vi "Forebrain - Bill.vi"() -> ()   [LabVIEW 2012]
doc: "This VI contrains the Forebrain within the Olin Robot Architecture. It must be run first to load the appropriate mission definition files. It contains a finite state machine built around a tabbed Operator interface that will guide an operator through the startup, run shutdown mission sequence. After running it, run the Midbrain and Hindbrain VIS."
panel:
  out "Number Waypoints":i32
  out "NXT String Sent":string="$B^"
  in  "Soft E-Stop":bool
  out "NXT String Received":string
  out "return count":u32
  out "error out":errorcluster
  in  "error in 2":errorcluster
  out "Desired \nVelocity":i16=5
  out "Local\nHeading":i16=90
  out "Ycurrent":dbl format="%#_3g"
  out "Xcurrent":dbl format="%#_3g"
  out "Ystart":dbl
  out "Xstart":dbl
  in  "error in":errorcluster
  out "Robot Live":bool
  in  "E-Stop":bool
  in  "Tab":T1(tab)
  out "MissionTime (Min)":dbl(knob) scale=0.0..10.0
  out "LidarDist":i16
  out "IR Index":i32
  out "BatteryLevel":dbl(slide) scale=6.0..9.0
  out "String Received":string
  out "Send String":string="$B^"
  in  "VISA resource name":refnum<visa-resource-name>="COM6"
  in  "Mode":i16 min=0 max=99 step=1
  in  "Desired Vel":i16(slide)=7 scale=0.0..14.0
  in  "Local Head":i16(slide)=7 scale=0.0..14.0
  out "StartMissionMap":picture
  out "MapDARCheck":picture
  in  "RunRobot":bool
  in  "Tug letter":string="G"
  out "Tug X":i32
  out "Tug Y":i32
  out "Tug H":i32
  out "BS Time Out?":bool
  out "Buoy locations":cluster{"regular expression":string, i32, i32}[](array[cluster])
  out "Valid ?":bool
  out "Battery\nVolts":i16
  out "Base Station data rec'd":string
  out "udp rate":bool
  out "CollisionWarning":bool
  out "DebugMapDAR":picture
  in  "MapDAR Control":T2={"NumberOfBeams"=180, "SensorRange"=500.0, "Noise (0.1 to 1)"=0.0} {"Noise (0.1 to 1)" min=0.0 max=1.0 step=0.1; "SensorRange" min=500.0 max=1500.0 step=100.0; "NumberOfBeams" min=36 max=360 step=2}
  out "MapDAR Data (r:pixel b:degrees)":cluster{"Range":dbl, "Bearing":dbl}[](array[cluster])
  in  "Stop DebugSENSE":bool
  out "MissionMap":picture
  out "Tug position":T3
  out "initialized MDF":T4(array[cluster])
  out "Way Point Index":i32
  out "InitialWaypoint":cluster{"X":i16, "Y":i16}
  in  "Pen Color":u32(colorbox)=15671808
  in  "Select Pen Attributes":T5={"Width"=1, "Style"=enum."Solid"}
  out "Draw??":bool
  in  "WhereAmI?FromBase":T6
  out "(xr,yr)":cluster{"X":dbl, "Y":dbl}
  in  "RobotPosition":T3 {"xrobot" min=0.0 max=1177.0 step=10.0; "yrobot" min=0.0 max=850.0 step=10.0; "heading" min=0.0 max=7.0 step=0.1}
  out "MDF_Original":T4(array[cluster])
  out "WhatAroundMeMap?":cluster{"T":dbl, "Range":dbl, "Bearing":dbl}[](array[cluster])
  out "WayPointAct":dbl[](array[numeric])
  out "SteerAngle":dbl
  out "MissionDefFile":picture
  out "MDF":T4(array[cluster])
  in  "Select Your Behavior":T7(ring)
  out "No. of Waypoints":i32
  in  "Exit Planning":bool
  in  "BoatSpeed for Leg":dbl(slide)=8.0 min=-9.0 max=9.0 step=1.0 scale=0.0..14.0
  out "BuildMDF":bool
  out "WayPoint Position":cluster{"X":i32, "Y":i32}
  in  "Upper Midbrain Active":bool
  out "Send String to NXT":string="$B^"
  in  "Behavior Command":T7(ring)
  out "CollisionLight":bool
  out "Where? Manual":T6
  out "ActManual":bool
  in  "Manual Heading":i16(knob) min=0 max=14 step=1
  out "MWhat?":bool
  out "Where? 2":bool
  out "How? 2":bool
  in  "ManualModeStop":bool
  out "ManualModeMapDAR":picture
  out "ManualMissionMap":picture
  out "Battery":dbl(slide) scale=0.0..8.0
  in  "Manual Vel":dbl(slide) min=0.0 max=14.0 step=1.0 scale=0.0..14.0
  out "MissionTime":dbl(knob) scale=0.0..10.0
  out "Heading":cluster{dbl, dbl}(knob)={0.0, 34.390870865624734} scale=180.0..-179.0 scale format="%#_3g"
  out "Speed":i16(knob) scale=-6.0..6.0
  out "Current Behavior":T7(ring)
  out "Robot Position":cluster{"X":dbl, "Y":dbl} {"X" format="%#_3g"; "Y" format="%#_3g"}
  out "Ready":bool
  in  "Pause":bool
  in  "Rerun MDF":bool
  out "CollisionLight 2":bool
  out "Act":bool
  out "Neo-C":bool
  out "How?":bool
  out "What?":bool
  out "A Heading":cluster{dbl, dbl}(knob)={0.0, 34.390870865624734} scale=180.0..-180.0
  out "A Speed":dbl(knob) scale=-9.0..9.0
  out "AutoBattery":dbl(slide) scale=0.0..8.0
  out "AutoModeLIDAR":picture
  out "AutoMissionMap":picture
  in  "RunAutoMode":bool
  out "MissionTimeAuto":dbl(knob) scale=0.0..60.0
  out "Where?":bool
  out "Current Waypoint":dbl
  in  "Manual Override":bool
  in  "Destinations Array":i64[][](array[numeric])
  out "BAM Mission Map":picture
  in  "Pixel Y Goal":dbl
  in  "Pixel X Goal":dbl
  out "Pixel X":dbl
  out "Pixel Y":dbl
  out "Direction":dbl
  out "Base Station String":string
  out "Battery Level":dbl
  in  "Heading":i16(knob)=7
  in  "Velocity":i16(slide)=7 scale=0.0..14.0
  # "To run\nrobot,\nclick\narrow\nabove\n\nRun Robot button must be on"
  # "Operation Directions\n\n1)Click on Startup&\nShutdown tab.\n2) Click on Run \nArrow on menubar.\nRun Forebrain,\nvis from the project\nexplorer.\n3) Select a mssion \nmap file when asked.\n4) Check robot is \nfully operational on\nStartup tab.\n5) Debug with debug\ntabs as required.\n6) Select ManualMode\ntab and test drive \nrobot.\n7) Select PlanMission\ntab and set up \nmission.\n8) Go to AutoMode\ntab and run mission."
  # "Turns off drive\nmotors"
  # "Enter Olin Test  Pool"
  # "Xbee Com Port"
  # "xBee\"Send String\" (mode, desired velocity, local heading)"
  # "(Type in Tug Letter  L T G P  (look at boat cradle)"
  # "Should be on to\nrun"
  # "BoatG,X,Y,H,BoatT,X,Y,H,BoatP,X,Y.H,BoatL,X,Y,H,BuoyA,X,Y,BuoyB,X,Y,BuoyC,X,Y,BuoyD,X,Y,Time(hours,Min,Sec)"
  # "To stop  program \nturn off here"
  # "Use this tab\nto explore\nLIDAR\ndata and \noperation"
  # "Set\nNumberOfBeams\nSensorRange\nNoise\nto\nview\nsimulated\nsensor\ndata"
  # "Turn Debug Sim \nto leave this\ntab--->"
  # "This tab will auto\nreturn to Startup \nin 2 seconds"
  # "Clean up interface and make more useful for debugging behaviors"
  # "Build out interface and make more useful for debugging act"
  # "This tab will auto\nreturn to Startup \nin 2 seconds"
  # "Directions:\n1) Select Robot Behavior for each mission leg.\n2) Select Robot Speed for leg.\n3) Click on robots current location for first waypoint.\n4) Hold down button and drag to next\nwaypoint. Click on next leg waypoint.\n5) Hold mouse button down and drag to \nnext waypoint. \n6) Click on next waypoint. Repeat for full mission.\n7) MDF will store up to 20 waypoints."
  # "Remember to\nset boat\nleg speed !"
  # "Please Adjust Scroll Barrs in Tug Off Mode to Prevent  Extra Lines Being Drawn"
  # "\"Send String\" (mode, desired velocity, local heading)"
  # "Press to stop and return to StartUp"
  # "Open MidBrain\nArbiter to see\nBrain Waves"
  # "AutoMode\nAutomatically \nReturns to \nStartUp Mode"
  # "Pixel coordinates for destinations."
  # "BoatG,X,Y,H,BoatT,X,Y,H,BoatP,X,Y.H,BoatL,X,Y,H,BuoyA,X,Y,BuoyB,X,Y,BuoyC,X,Y,BuoyD,X,Y,Time(hours,Min,Sec)"
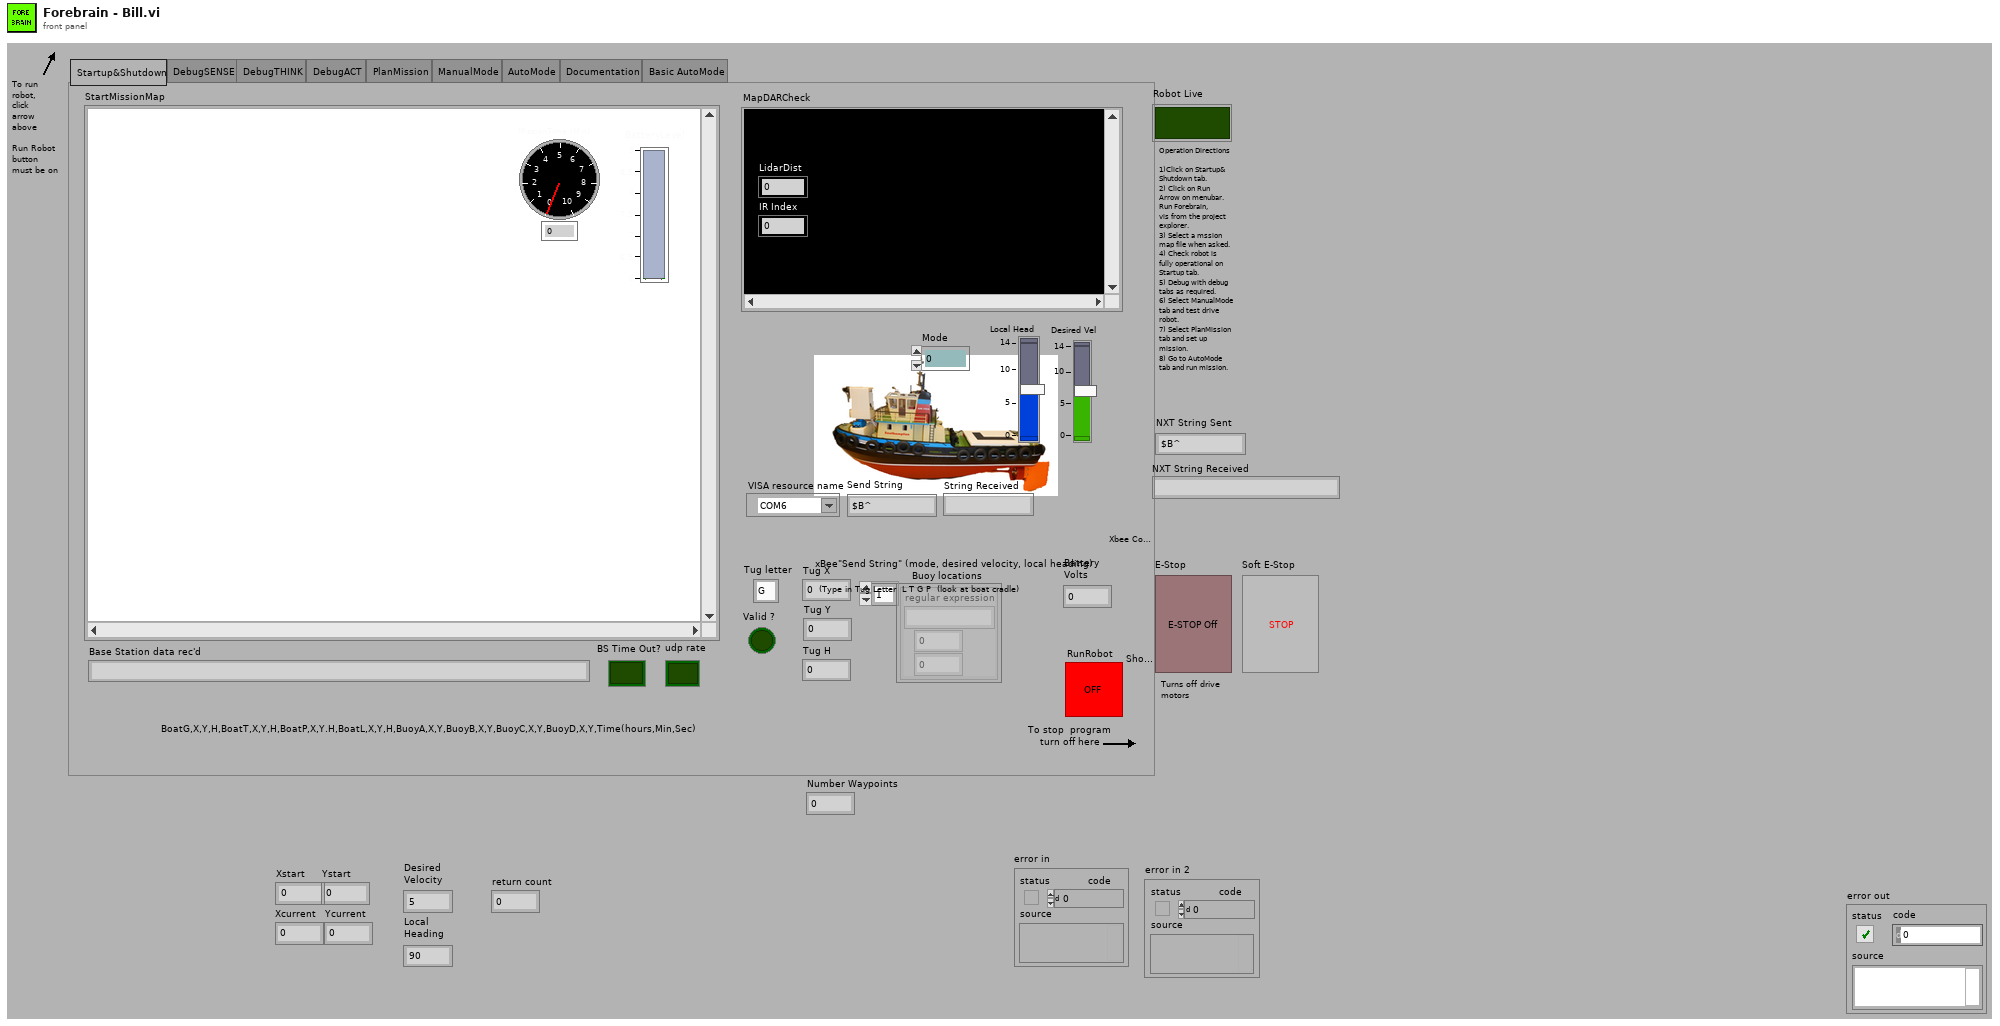
[diagram p1: front panel]
types:
  T1 = enum32{"Startup&Shutdown", "DebugSENSE", "DebugTHINK", "DebugACT", "PlanMission", "ManualMode", "AutoMode", "Documentation", "Basic AutoMode"}
  T2 = cluster{"NumberOfBeams":i32, "SensorRange":dbl, "Noise (0.1 to 1)":dbl}
  T3 = cluster{"xrobot":dbl, "yrobot":dbl, "heading":dbl}
  T4 = cluster{"Status":enum16{"Past", "Current", "Future"}, "x":dbl, "y":dbl, "z":dbl, "Vel":dbl, "Dwell Time":dbl, "BehCom":enum16{"Tug Off", "Manual Mode", "Goto WayPoint", "Back Up", "Circle", "Left Wall Follow", "Right Wall Follow", "Hunt"}, "Expand1":dbl, "Expand2":dbl, "Expand3":dbl}[]
  T5 = cluster{"Width":u16, "Style":enum32{"Solid", "Dash", "Dot", "DashDot", "DashDotDot"}}
  T6 = cluster{"T":dbl, "X":dbl, "Y":dbl, "Direction":dbl}
  T7 = enum16{"Tug Off", "Manual Mode", "Goto WayPoint", "Back Up", "Circle", "Left Wall Follow", "Right Wall Follow", "Hunt"}
  T8 = enum32{"Startup&Shutdown", "DebugSENSE", "DebugTHINK", "DebugACT", "PlanMission", "ManualMode", "AutoMode", "Documentation"}
  T9 = cluster{"VelCom":dbl, "BehCom":enum16{"OpenFieldTransit", "P-WallFollow", "S-WallFollow", "LaneFollow", "ManualMode"}}
  T10 = typedef "IMAQ Image.ctl" = refnum<image>
  T11 = typedef "imagedata.ctl" = cluster{"image type":i32, "image depth":i32, "image":u8[], "mask":u8[], "colors":u32[], "Rectangle":cluster{"left":i16, "top":i16, "right":i16, "bottom":i16}}
  T12 = cluster{"Status":enum16{"Past", "Current", "Future"}, "x":dbl, "y":dbl, "z":dbl, "Vel":dbl, "Dwell Time":dbl, "BehCom":enum16{"Tug Off", "Manual Mode", "Goto WayPoint", "Back Up", "Circle", "Left Wall Follow", "Right Wall Follow", "Hunt"}, "Expand1":dbl, "Expand2":dbl, "Expand3":dbl}
  T13 = typedef "LVMouseTypeDef.ctl" = cluster{"Mouse Position":cluster{"X":i32, "Y":i32}, "Mouse Modifiers":cluster{"Button Down":bool, "Shift Mod":bool, "Menu Mod":bool, "Option Mod":bool}}
  T14 = cluster{"regular expression":string, i32, i32, i32}
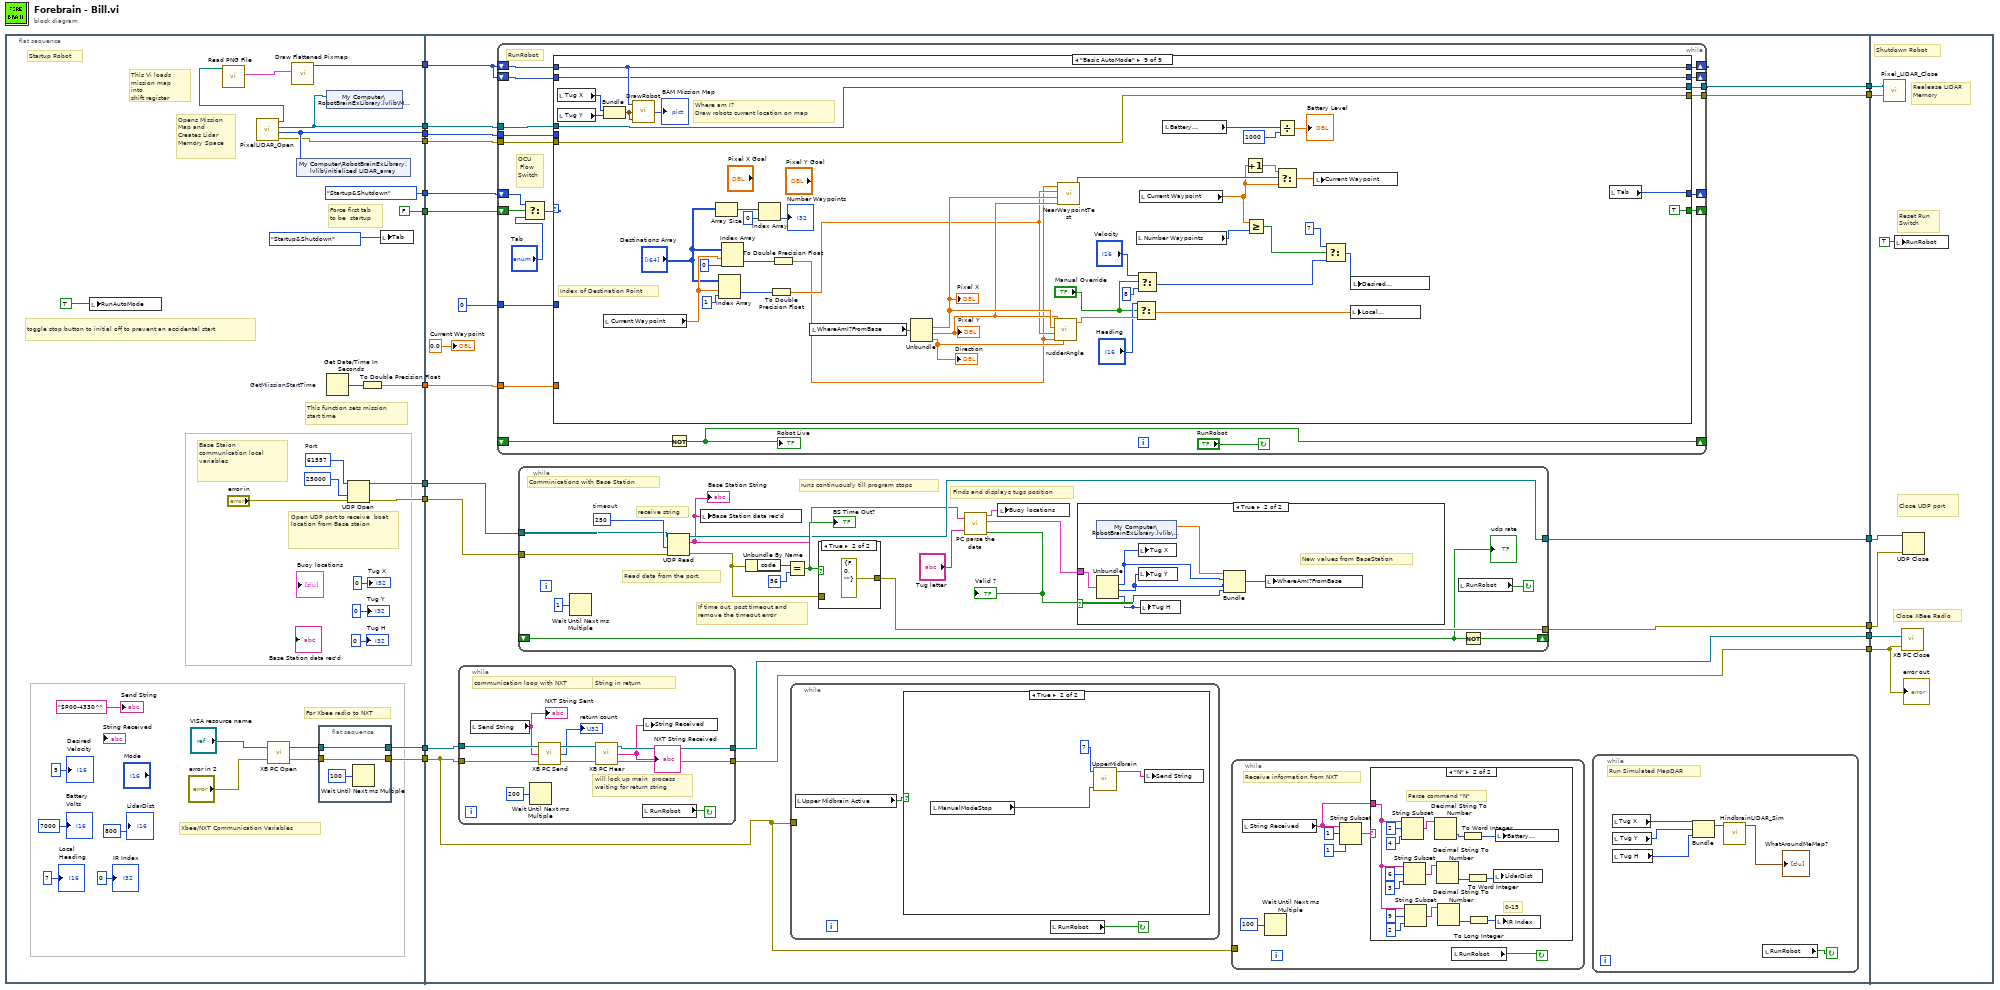
[diagram p0: block diagram]
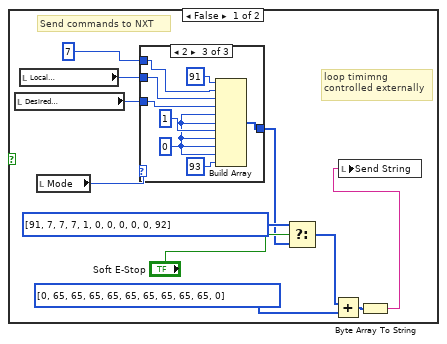
[diagram p3: hidden frame]
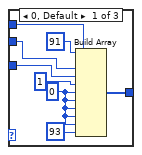
[diagram p4: hidden frame]
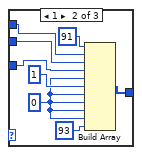
[diagram p5: hidden frame]
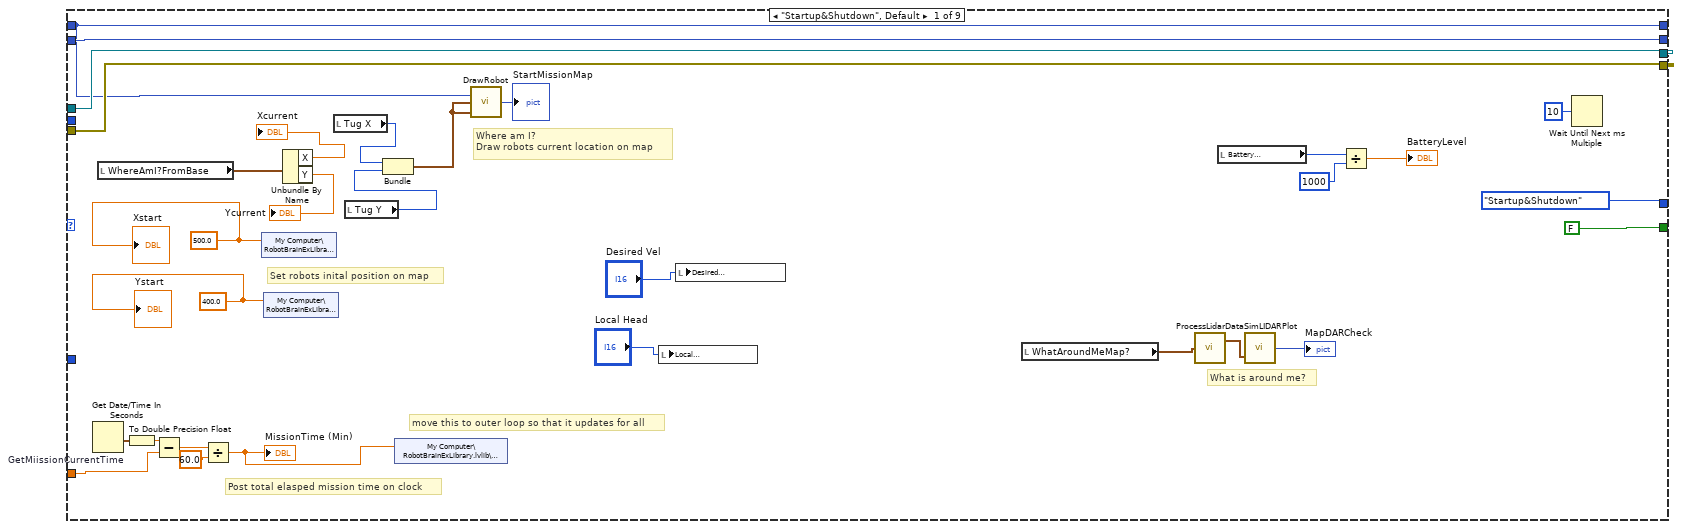
[diagram p8: hidden frame]
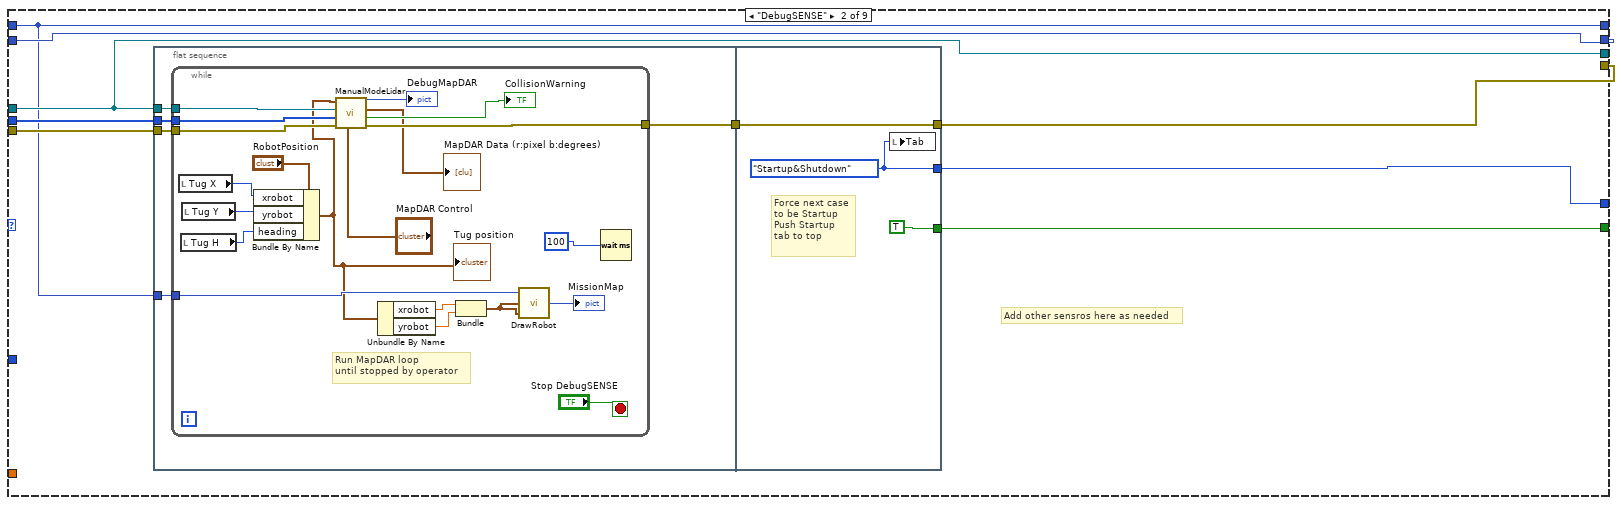
[diagram p9: hidden frame]
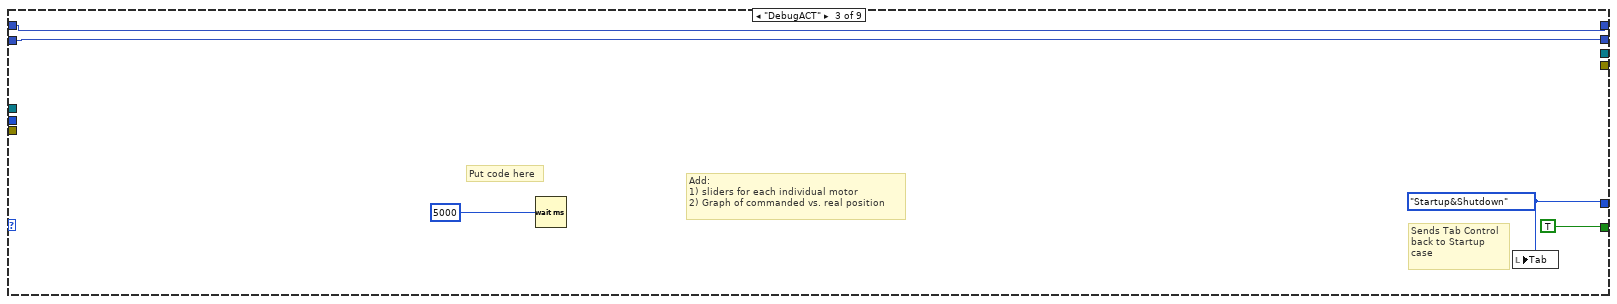
[diagram p10: hidden frame]
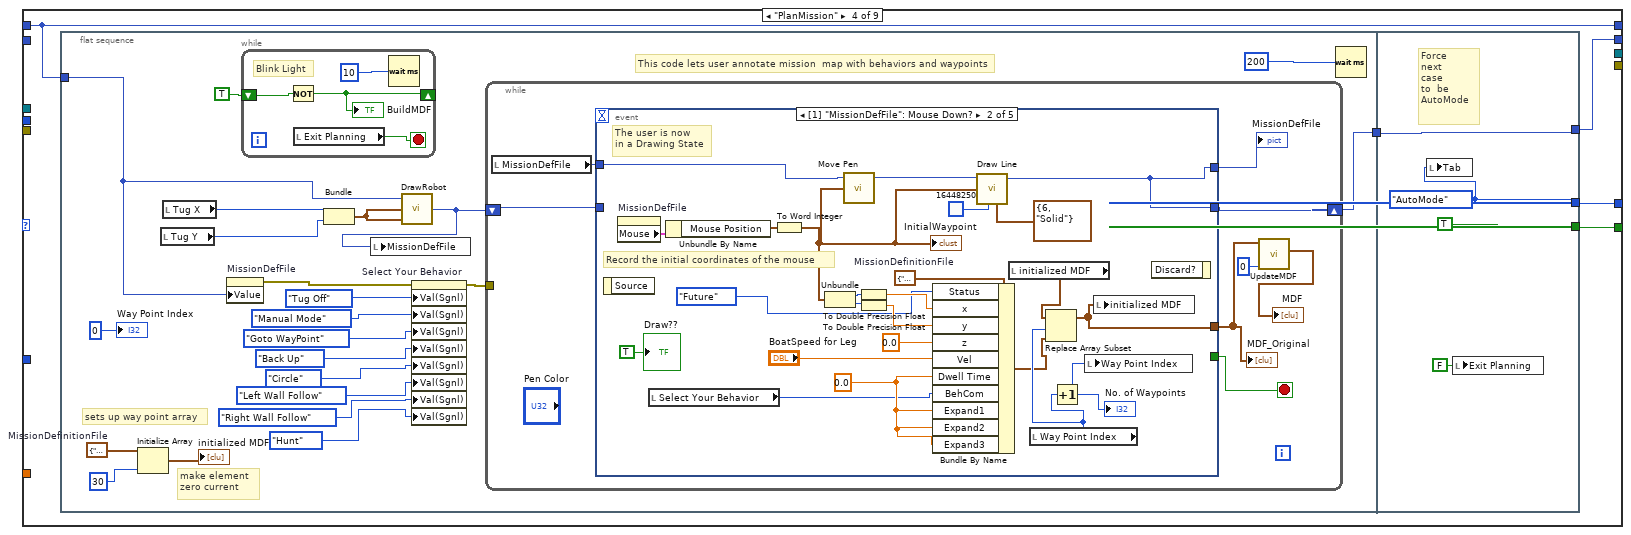
[diagram p11: hidden frame]
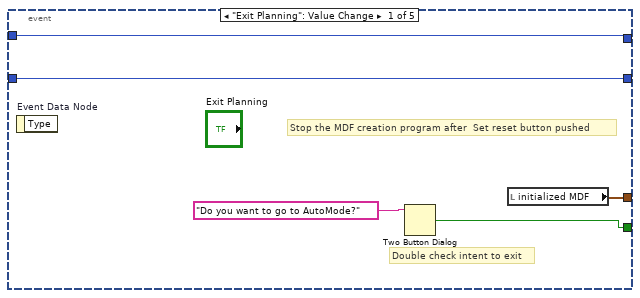
[diagram p12: hidden frame]
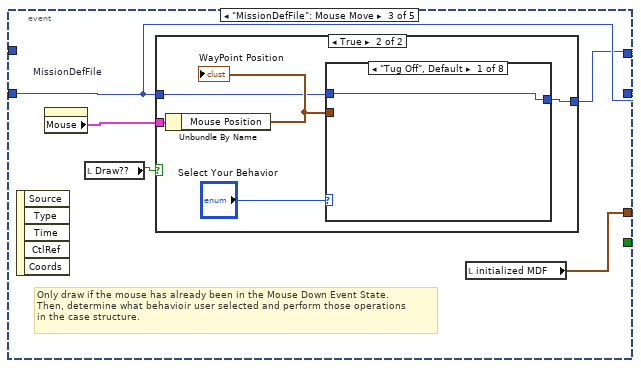
[diagram p13: hidden frame]
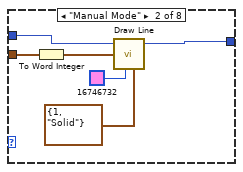
[diagram p15: hidden frame]
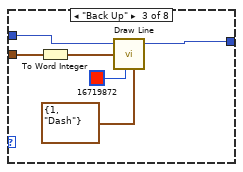
[diagram p16: hidden frame]
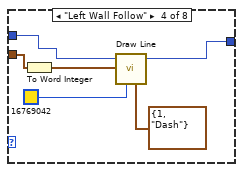
[diagram p17: hidden frame]
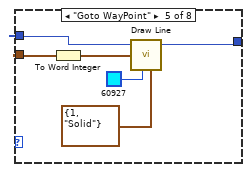
[diagram p18: hidden frame]
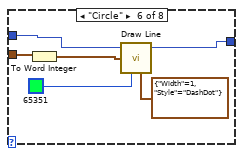
[diagram p19: hidden frame]
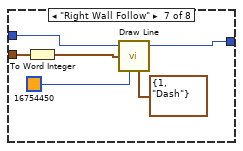
[diagram p20: hidden frame]
diagram:
  n1 = flat-sequence {
    tunnel: [w48] -> w17
    tunnel: [w47] -> w16
    tunnel: [w44] -> w15
    tunnel: [w46] -> w14
    tunnel: [w45] -> w13
    tunnel: [FALSE ("RunAutoMode")] -> w10
    tunnel: [T8."Startup&Shutdown" ("Tab")] -> w9
    tunnel: [w31] -> w8
    tunnel: [w30] -> w7
    tunnel: [w19] -> w6
    tunnel: [w18] -> w5
    tunnel: w17 -> [w71]
    tunnel: w16 -> [w70]
    tunnel: w15 -> [w69]
    tunnel: w14 -> [w68]
    tunnel: w13 -> [w67]
    tunnel: [w66] -> w12
    tunnel: [w65] -> w11
    tunnel: w10 -> [w64]
    tunnel: w9 -> [w63]
    tunnel: w8 -> [w58]
    tunnel: w7 -> [w57]
    tunnel: w6 -> [w62]
    tunnel: w5 -> [w59]
    tunnel: [w61] -> w4
    tunnel: [w60] -> w3
    tunnel: [w56] -> w2
    tunnel: [w55] -> w1
    tunnel: w12 -> [w662]
    tunnel: w11 -> [w661]
    tunnel: w4 -> [w660]
    tunnel: w3 -> [w659]
    tunnel: w2 -> [w658]
    tunnel: w1 -> [w657]
    frame #0 {
      w37 = u16 61557  # Port
      # "For Xbee radio to NXT"
      # "Xbee/NXT Communication Variables"
      # "Base Staion communication local variables"
      # "Open UDP port to receive  boat location from Base staion"
      # "Force first tab\nto be  startup"
      # "toggle stop button to initial off to prevent an accidental start"
      # "Opens Mission\nMap and\nCreates Lidar\nMemory Space"
      # "This function sets mission \nstart time"
      # "This Vi loads\nmission map into \nshift register"
      # "Startup Robot"
      n2 = local write "RunAutoMode"(TRUE ("RunAutoMode")) -> ()
      n3 = call "PixelLIDAR_Open.vi"() -> ("error out"=w45:errorcluster, "initialized LIDAR\narray"=w46:i32[], "MDF Image"=w44:T10, "MissionMap"=w39:path)  [unwired: 2 in]
      n4 = call <vilib>:"Read PNG File.vi"("path to PNG file"=w39) -> ("image data"=w38:T11)  [unwired: 8 in, 2 out]
      n5 = call "XB PC Open.vi"("error in (no error)"="error in 2", "VISA resource name"="VISA resource name") -> ("error out"=w22:errorcluster, "VISA resource name out"=w23:refnum<visa-resource-name>)
      n6 = call <vilib>:"Draw Flattened Pixmap.vi"("image data"=w38) -> ("new picture"=w47:picture)  [unwired: 8 in]
      n7 = shared-variable "My Computer\\RobotBrainExLibrary.lvlib\\initialized LIDAR_array"(w46) -> ()  [unwired: 1 in, 1 out]
      n8 = flat-sequence {
        tunnel: w23 -> [w50]
        tunnel: w22 -> [w51]
        tunnel: [w51] -> w18
        tunnel: [w50] -> w19
        frame #0 {
          n9 = Wait Until Next ms Multiple(millisecond multiple=u32 100) -> ()  [unwired: 1 out]
        }
      }
      n10 = shared-variable "My Computer\\RobotBrainExLibrary.lvlib\\MDF Image"(w44) -> ()  [unwired: 1 in, 1 out]
      n11 = Get Date/Time In Seconds "GetMiissionStartTime"() -> (seconds since 1Jan1904=w49:timestamp)
      n12 = UDP Open(8:"error in", 9:25000 ("timeout ms (25000)"), 11:w37) -> (port=w31:refnum<k16>, 0:w30:errorcluster)  [unwired: 2 in, 1 out]
      n13 = To Double Precision Float(number=w49) -> (double precision float=w48:dbl)
      n14 = local write "Tab"(T8."Startup&Shutdown" ("Tab")) -> ()
      "Tug X" <- 0 ("Tug X")
      "Tug Y" <- 0 ("Tug Y")
      "Tug H" <- 0 ("Tug H")
      "Battery\nVolts" <- i16 7000 ("Battery\nVolts")
      "LidarDist" <- i16 800 ("Dist")
      "IR Index" <- 0 ("IR Index")
      "Local\nHeading" <- i16 7 ("Local\nHeading")
      "Desired \nVelocity" <- i16 5 ("Desired \nVelocity")
      "Send String" <- "$P00-4330^"
    }
    frame #1 {
      n15 = while {
        tunnel: w62 -> [w150]
        tunnel: w59 -> [w149]
        tunnel: [w146] -> w60
        tunnel: [w145] -> w61
        stop <- w144 continue-if-true
        # "will lock up main  process\nwaiting for return string"
        # "communication loop with NXT"
        # "send a string to the NXT and receive a String in return"
        n16 = local read "Send String"() -> (w142:string)
        "NXT String Sent" <- w142
        n17 = Wait Until Next ms Multiple(millisecond multiple=u32 200) -> ()  [unwired: 1 out]
        n18 = call "XB PC Send.vi"("error in (no error)"=w149, "String"=w142, "VISA resource name"=w150) -> ("error out"=w148:errorcluster, "return count"=→"return count":u32, "VISA resource name out"=w147:refnum<visa-resource-name>)
        n19 = call "XB PC Hear.vi"("VISA resource name"=w147, "error in (no error)"=w148) -> ("VISA resource name out"=w145:refnum<visa-resource-name>, "String Received"=w141:string, "error out"=w146:errorcluster)
        "NXT String Received" <- w141
        n20 = local read "RunRobot"() -> (w144:bool)
        n21 = local write "String Received"(w141) -> ()
      }
      n22 = while {
        shift-right: [w179] -> _
        shift-left: _ -> [w195]
        shift-right: [w194] -> _
        shift-left: w63 -> [w193]
        shift-right: [w190] -> _
        shift-left: w64 -> [w189]
        tunnel: w71 -> [w188]
        shift-right: [w178] -> _
        shift-left: w70 -> [w187]
        shift-right: [w185] -> _
        shift-left: w70 -> [w186]
        tunnel: w69 -> [w184]
        tunnel: w68 -> [w183]
        tunnel: w67 -> [w182]
        tunnel: [w181] -> w66
        tunnel: [w180] -> w65
        tunnel: 0 -> [w177]
        stop <- "RunRobot" continue-if-true
        # "RunRobot"
        # "OCU\n Flow\nSwitch"
        n23 = Select(t=w193, s=w189, f="Tab") -> (s? t:f=w191:T1)
        n24 = case shown="\"Basic AutoMode\"" w191 {
          selector: w191 -> [_ _ _ _ _ w515 _ _ _]
          tunnel: [T8."Startup&Shutdown" ("Tab") w231 w266 w273 w440 w516 T8."Startup&Shutdown" ("Tab") w612 w644] -> w194
          tunnel: [FALSE ("s") w230 TRUE ("s") w272 w441 w514 FALSE ("s") TRUE ("s") TRUE ("s")] -> w190
          tunnel: w188 -> [w220 _ _ _ w438 w512 _ _ _]
          tunnel: w187 -> [w197 w227 w265 w269 w436 w509 w605 w610 w650]
          tunnel: w186 -> [w219 w228 w264 _ w437 w511 w604 w609 w649]
          tunnel: [w219 w228 w264 w270 w437 w511 w604 w609 w649] -> w185
          tunnel: w184 -> [w218 w229 _ _ _ _ _ _ w645]
          tunnel: w183 -> [_ w235 _ _ _ _ _ _ _]
          tunnel: w182 -> [w217 w234 _ _ _ _ _ _ w642]
          tunnel: [w218 w229 _ _ _ _ _ _ w645] -> w181
          tunnel: [w217 w233 _ _ _ _ _ _ w642] -> w180
          tunnel: [w197 w227 w265 w269 w436 w509 w605 w610 w650] -> w178
          tunnel: w177 -> [_ _ _ _ _ _ _ _ _]
          frame "Startup&Shutdown", Default {
            w209 = 400.0 ("Ystart")
            w210 = 500.0 ("Xstart")
            # "move this to outer loop so that it updates for all"
            # "Where am I?\nDraw robots current location on map"
            # "Post total elasped mission time on clock"
            # "What is around me?"
            # "Set robots inital position on map"
            n25 = Get Date/Time In Seconds "GetMiissionCurrentTime"() -> (seconds since 1Jan1904=w224:timestamp)
            n26 = local read "WhereAmI?FromBase"() -> (w198:T6)
            n27 = To Double Precision Float(number=w224) -> (double precision float=w223:dbl)
            n28 = Subtract(x=w223, y=w220) -> (x-y=w222:dbl)
            n29 = Divide(x=w222, y=60.0) -> (x/y=w216:dbl)
            "MissionTime (Min)" <- w216
            n30 = shared-variable "My Computer\\RobotBrainExLibrary.lvlib\\Xstart"(w210) -> ()  [unwired: 1 in, 1 out]
            n31 = shared-variable "My Computer\\RobotBrainExLibrary.lvlib\\Ystart"(w209) -> ()  [unwired: 1 in, 1 out]
            n32 = Unbundle By Name(w198) -> ("X"=→"Xcurrent":dbl, "Y"=→"Ycurrent":dbl)
            n33 = local read "Tug X"() -> (w208:i32)
            n34 = local read "Tug Y"() -> (w207:i32)
            n35 = Bundle("Tug X"=w208, "Tug Y"=w207) -> (w213:cluster{"Tug X":i32, "Tug Y":i32})  [unwired: 1 in]
            n36 = shared-variable "My Computer\\RobotBrainExLibrary.lvlib\\MissionTime"(w216) -> ()  [unwired: 1 in, 1 out]
            n37 = call "DrawRobot.vi"("(xr,yr) old"=w213, "(xr,yr) new"=w213, "2D Picture"=w197) -> ("new picture"=→"StartMissionMap":picture)
            n38 = local write "Local\nHeading"("Local Head") -> ()
            n39 = local write "Desired \nVelocity"("Desired Vel") -> ()
            n40 = local read "WhatAroundMeMap?"() -> (w199:cluster{"T":dbl, "Range":dbl, "Bearing":dbl}[])
            n41 = call "ProcessLidarData.vi"("WhatAroundMe?MM"=w199) -> ("data array [mag, phase (deg)]"=w214:cluster{"magnitude":dbl, "phase":dbl}[])  [unwired: 1 out]
            n42 = local read "Battery\nVolts"() -> (w204:i16)
            n43 = call "SimLIDARPlot.vi"("data array [mag, phase (deg)]"=w214) -> ("SONAR"=→"MapDARCheck":picture)  [unwired: 1 in]
            n44 = Divide(x=w204, y=i16 1000) -> (x/y=→"BatteryLevel":dbl)
            n45 = Wait Until Next ms Multiple(millisecond multiple=u32 10) -> ()  [unwired: 1 out]
            "Xstart" <- w210
            "Ystart" <- w209
          }
          frame "DebugSENSE" {
            # "Add other sensros here as needed"
            n46 = flat-sequence {
              tunnel: w235 -> [w240]
              tunnel: w234 -> [w239]
              tunnel: w229 -> [w238]
              tunnel: [w237] -> w232
              tunnel: w227 -> [w236]
              tunnel: [w263] -> w233
              tunnel: w232 -> [w263]
              tunnel: [w262] -> w231
              tunnel: [TRUE ("s")] -> w230
              frame #0 {
                n47 = while {
                  tunnel: w240 -> [w260]
                  tunnel: w239 -> [w259]
                  tunnel: w238 -> [w258]
                  tunnel: [w257] -> w237
                  tunnel: w236 -> [w251]
                  stop <- "Stop DebugSENSE" stop-if-true
                  # "Run MapDAR loop\nuntil stopped by operator"
                  n48 = local read "Tug X"() -> (w245:i32)
                  n49 = local read "Tug H"() -> (w246:i32)
                  n50 = local read "Tug Y"() -> (w244:i32)
                  n51 = Bundle By Name(cluster="RobotPosition", "xrobot"=w245, "yrobot"=w244, "heading"=w246) -> (w242:T3)
                  "Tug position" <- w242
                  n52 = call "ManualModeLidar.vi"("LIDARControl"="MapDAR Control", "error in"=w259, "initialized \nsonar ray\narray"=w260, "MDF Image"=w258, "SubPosition"=w242) -> ("error out"=w257:errorcluster, "Collision\nWarning"=→"CollisionWarning":bool, "LIDAR Data (r:pixel b:degrees)"=→"MapDAR Data (r:pixel b:degrees)":cluster{"Range":dbl, "Bearing":dbl}[], "LIDAR"=→"DebugMapDAR":picture)  [unwired: 1 in]
                  n53 = Unbundle By Name(w242) -> ("xrobot"=w249:dbl, "yrobot"=w248:dbl)
                  n54 = Bundle("xrobot"=w249, "yrobot"=w248) -> (w241:cluster{"xrobot":dbl, "yrobot":dbl})  [unwired: 1 in]
                  n55 = call "DrawRobot.vi"("(xr,yr) old"=w241, "(xr,yr) new"=w241, "2D Picture"=w251) -> ("new picture"=→"MissionMap":picture)
                  n56 = Wait (ms)(milliseconds to wait=u32 100) -> ()  [unwired: 1 out]
                }
              }
              frame #1 {
                w262 = T8."Startup&Shutdown" ("Tab")
                # "Force next case\nto be Startup\nPush Startup\ntab to top"
                n57 = local write "Tab"(w262) -> ()
              }
            }
          }
          frame "DebugACT" {
            w266 = T8."Startup&Shutdown" ("Tab")
            # "Add:\n1) sliders for each individual motor\n2) Graph of commanded vs. real position"
            # "Put code here"
            # "Sends Tab Control\nback to Startup\ncase"
            n58 = Wait (ms)(milliseconds to wait=u32 5000) -> ()  [unwired: 1 out]
            n59 = local write "Tab"(w266) -> ()
          }
          frame "PlanMission" {
            n60 = flat-sequence {
              tunnel: [w294] -> w271
              tunnel: w269 -> [w287]
              tunnel: [w434] -> w273
              tunnel: [TRUE ("s")] -> w272
              tunnel: w271 -> [w433]
              tunnel: [w433] -> w270
              frame #0 {
                w285 = T12 {"Status"=enum."Future", "x"=0.0, "y"=0.0, "z"=0.0, "Vel"=0.0, "Dwell Time"=0.0, "BehCom"=enum."Tug Off", "Expand1"=0.0, "Expand2"=0.0, "Expand3"=0.0}  # MissionDefinitionFile
                # "make element \nzero current"
                # "sets up way point array"
                # "This code lets user annotate mission  map with behaviors and waypoints"
                n61 = Initialize Array ("Initialize WaypointArray")(w285, 30 ("dimension size")) -> (→"initialized MDF":T4)
                n62 = local read "Tug Y"() -> (w282:i32)
                n63 = local read "Tug X"() -> (w283:i32)
                n64 = property on="MissionDefFile" class="Pict"("Value"=w287) -> (error out=w292:errorcluster)  [unwired: 2 in, 1 out]
                n65 = while {
                  shift-right: [w298] -> _
                  shift-left: TRUE -> [w299]
                  stop <- w297 stop-if-true
                  # "Blink Light"
                  n66 = Not(x=w299) -> (.not. x?=w298:bool)
                  "BuildMDF" <- w298
                  n67 = local read "Exit Planning"() -> (w297:bool)
                  n68 = Wait (ms)(milliseconds to wait=u32 10) -> ()  [unwired: 1 out]
                }
                n69 = Bundle("Tug X"=w283, "Tug Y"=w282) -> (w288:cluster{"Tug X":i32, "Tug Y":i32})  [unwired: 1 in]
                n70 = call "DrawRobot.vi"("(xr,yr) old"=w288, "(xr,yr) new"=w288, "2D Picture"=w287) -> ("new picture"=w286:picture)
                n71 = local write "MissionDefFile"(w286) -> ()
                n72 = property on="Select Your Behavior" class="Enum (strict)"(error in=w292, "Val(Sgnl)"=T7."Tug Off" ("Value (Signaling)"), "Val(Sgnl)"=T7."Manual Mode" ("Value (Signaling)"), "Val(Sgnl)"=T7."Goto WayPoint" ("Value (Signaling)"), "Val(Sgnl)"=T7."Back Up" ("Value (Signaling)"), "Val(Sgnl)"=T7."Circle" ("Value (Signaling)"), "Val(Sgnl)"=T7."Left Wall Follow" ("Value (Signaling)"), "Val(Sgnl)"=T7."Right Wall Follow" ("Value (Signaling)"), "Val(Sgnl)"=T7."Hunt" ("Value (Signaling)")) -> (error out=w293:errorcluster)  [unwired: 1 in, 1 out]
                n73 = while {
                  shift-right: [w306] -> w294
                  shift-left: w286 -> [w307]
                  tunnel: w293 -> [_]
                  stop <- w305 stop-if-true
                  n74 = local read "MissionDefFile"() -> (w304:picture)
                  n75 = event shown="[1] \"MissionDefFile\": Mouse Down?" {
                    selector: _ -> [_ _ _ _ _]
                    dyn-events: _ -> [_ _ _ _ _]
                    timeout: _ -> [_ _ _ _ _]
                    tunnel: [w310 w318 w338 w391 w429] -> w306
                    tunnel: w307 -> [w310 _ w338 w391 _]
                    tunnel: [w311 _ _ _ _] -> w305
                    tunnel: [w309 w333 w339 w393 w430] -> w301
                    tunnel: w304 -> [w308 w319 _ w392 w429]
                    tunnel: [w308 w318 w337 w392 w429] -> w303
                    event "Exit Planning": Value Change {
                      # "Double check intent to exit"
                      # "Stop the MDF creation program after  Set reset button pushed"
                      n76 = event-data "Event Data Node"() -> ()  [unwired: 1 in, 1 out]
                      n77 = Two Button Dialog(message="Do you want to go to AutoMode?") -> (T button?=w311:bool)  [unwired: 2 in]
                      n78 = local read "initialized MDF"() -> (w309:T4)
                    }
                    event "MissionDefFile": Mouse Down? {
                      w317 = T12 {"Status"=enum."Future", "x"=0.0, "y"=0.0, "z"=0.0, "Vel"=0.0, "Dwell Time"=0.0, "BehCom"=enum."Tug Off", "Expand1"=0.0, "Expand2"=0.0, "Expand3"=0.0}  # MissionDefinitionFile
                      w327 = 0.0 ("Dwell Time")
                      # "Record the initial coordinates of the mouse"
                      # "The user is now\nin a Drawing State"
                      n79 = event-data() -> ()  [unwired: 1 in, 1 out]
                      n80 = property on="MissionDefFile" class="Pict"() -> ("Mouse"=w336:T13)  [unwired: 2 in, 2 out]
                      n81 = local read "Select Your Behavior"() -> (w314:T7)
                      n82 = Unbundle By Name(w336) -> ("Mouse Position"=w334:cluster{"X":i32, "Y":i32})
                      n83 = To Word Integer(number=w334) -> (16bit integer=w322:cluster{"X":i16, "Y":i16})
                      "InitialWaypoint" <- w322
                      n84 = Unbundle(w322) -> ("X"=w331:i16, "Y"=w330:i16)
                      n85 = call <vilib>:"Move Pen.vi"("new position"=w322, "picture"=w319) -> ("new picture"=w323:picture)  [unwired: 3 in]
                      n86 = To Double Precision Float(number=w331) -> (double precision float=w329:dbl)
                      n87 = To Double Precision Float(number=w330) -> (double precision float=w328:dbl)
                      n88 = Bundle By Name(cluster=w317, "Status"=enum16{"Past", "Current", "Future"}."Future", "x"=w329, "y"=w328, "z"=0.0, "Vel"="BoatSpeed for Leg", "Dwell Time"=w327, "BehCom"=w314, "Expand1"=w327, "Expand2"=w327, "Expand3"=w327) -> (w313:T12)
                      n89 = call <vilib>:"Draw Line.vi"("picture"=w323, "end point"=w322, "color(black)"=u32 16448250, "pen"=T5 {"Width"=6, "Style"=enum."Solid"}) -> ("new picture"=w318:picture)  [unwired: 5 in]
                      n90 = local read "initialized MDF"() -> (w332:T4)
                      n91 = local read "Way Point Index"() -> (w315:i32)
                      n92 = Replace Array Subset(array=w332, new element=w313, index=w315) -> (w333:T4)
                      n93 = Increment(x=w315) -> (x+1=w335:i32)
                      "No. of Waypoints" <- w335
                      n94 = local write "Way Point Index"(w335) -> ()
                      n95 = local write "initialized MDF"(w333) -> ()
                      n96 = event-data() -> ()  [unwired: 2 in, 1 out]
                      "Draw??" <- TRUE ("Draw??")
                    }
                    event "MissionDefFile": Mouse Move {
                      # "Only draw if the mouse has already been in the Mouse Down Event State.\nThen, determine what behavioir user selected and perform those operations\nin the case structure."
                      n97 = event-data() -> ()  [unwired: 1 in, 5 out]
                      n98 = property on="MissionDefFile" class="Pict"() -> ("Mouse"=w341:T13)  [unwired: 2 in, 2 out]
                      n99 = local read "Draw??"() -> (w340:bool)
                      n100 = case shown="True" w340 {
                        tunnel: w341 -> [_ w347]
                        tunnel: w338 -> [w342 w343]
                        tunnel: [w342 w344] -> w337
                        frame False {
                        }
                        frame True {
                          n101 = Unbundle By Name(w347) -> ("Mouse Position"=w345:cluster{"X":i32, "Y":i32})
                          "WayPoint Position" <- w345
                          n102 = case shown="\"Tug Off\", Default" "Select Your Behavior" {
                            tunnel: w345 -> [_ w353 w359 w362 w368 w373 w379 w385]
                            tunnel: [w348 w354 w360 w364 w367 w374 w380 w386] -> w344
                            tunnel: w343 -> [w348 w352 w356 w365 w369 w375 w381 w387]
                            frame "Tug Off", Default {
                            }
                            frame "Manual Mode" {
                              n103 = To Word Integer(number=w353) -> (16bit integer=w349:cluster{"X":i16, "Y":i16})
                              n104 = call <vilib>:"Draw Line.vi"("picture"=w352, "end point"=w349, "color(black)"=u32 16746732, "pen"=T5 {"Width"=1, "Style"=enum."Solid"}) -> ("new picture"=w354:picture)  [unwired: 5 in]
                            }
                            frame "Back Up" {
                              n105 = To Word Integer(number=w359) -> (16bit integer=w355:cluster{"X":i16, "Y":i16})
                              n106 = call <vilib>:"Draw Line.vi"("picture"=w356, "end point"=w355, "color(black)"=u32 16719872, "pen"=T5 {"Width"=1, "Style"=enum."Dash"}) -> ("new picture"=w360:picture)  [unwired: 5 in]
                            }
                            frame "Left Wall Follow" {
                              n107 = To Word Integer(number=w362) -> (16bit integer=w363:cluster{"X":i16, "Y":i16})
                              n108 = call <vilib>:"Draw Line.vi"("picture"=w365, "end point"=w363, "color(black)"=u32 16769042, "pen"=T5 {"Width"=1, "Style"=enum."Dash"}) -> ("new picture"=w364:picture)  [unwired: 5 in]
                            }
                            frame "Goto WayPoint" {
                              n109 = To Word Integer(number=w368) -> (16bit integer=w370:cluster{"X":i16, "Y":i16})
                              n110 = call <vilib>:"Draw Line.vi"("picture"=w369, "end point"=w370, "color(black)"=u32 60927, "pen"=T5 {"Width"=1, "Style"=enum."Solid"}) -> ("new picture"=w367:picture)  [unwired: 5 in]
                            }
                            frame "Circle" {
                              n111 = To Word Integer(number=w373) -> (16bit integer=w378:cluster{"X":i16, "Y":i16})
                              n112 = call <vilib>:"Draw Line.vi"("picture"=w375, "end point"=w378, "color(black)"=u32 65351, "pen"=T5 {"Width"=1, "Style"=enum."DashDot"}) -> ("new picture"=w374:picture)  [unwired: 5 in]
                            }
                            frame "Right Wall Follow" {
                              n113 = To Word Integer(number=w379) -> (16bit integer=w384:cluster{"X":i16, "Y":i16})
                              n114 = call <vilib>:"Draw Line.vi"("picture"=w381, "end point"=w384, "color(black)"=u32 16754450, "pen"=T5 {"Width"=1, "Style"=enum."Dash"}) -> ("new picture"=w380:picture)  [unwired: 5 in]
                            }
                            frame "Hunt" {
                              n115 = To Word Integer(number=w385) -> (16bit integer=w388:cluster{"X":i16, "Y":i16})
                              n116 = call <vilib>:"Draw Line.vi"("picture"=w387, "end point"=w388, "color(black)"=u32 16720896, "pen"=T5 {"Width"=1, "Style"=enum."DashDotDot"}) -> ("new picture"=w386:picture)  [unwired: 5 in]
                            }
                          }
                        }
                      }
                      n117 = local read "initialized MDF"() -> (w339:T4)
                    }
                    event "Select Your Behavior": Value Change {
                      # "When the user selects a new operation, we disable certain controls that aren't relevant to\nthe operation that the user is performing."
                      n118 = event-data() -> ("NewVal"=w396:T7)  [unwired: 1 in]
                      n119 = property on="Select Pen Attributes" class="Clust (strict)"() -> ("Controls[]"=w395:refnum<vi>[])  [unwired: 2 in, 2 out]
                      n120 = case shown="\"Manual Mode\"" w396 {
                        tunnel: w395 -> [w400 w401 w405 w409 w413 w417 w421 w425]
                        tunnel: "Select Pen Attributes" -> [_ _ _ _ _ _ _ _]
                        frame "Manual Mode" {
                          # "All attributes are valid for this\noperation."
                          n121 = Index Array "Index Array"(array=w400, index=1) -> (element=w398:refnum<vi>)
                          n122 = property on="Property Node" class="Ctl"(reference=w398, "Disabled"=u8 0) -> ()  [unwired: 1 in, 2 out]
                        }
                        frame "Back Up" {
                          # "All attributes are valid for this\noperation."
                          n123 = Index Array(array=w401, index=1) -> (element=w403:refnum<vi>)
                          n124 = property class="Ctl"(reference=w403, "Disabled"=u8 0) -> ()  [unwired: 1 in, 2 out]
                        }
                        frame "Tug Off" {
                          # "All attributes are valid for this\noperation."
                          n125 = Index Array "Index Array"(array=w405, index=1) -> (element=w407:refnum<vi>)
                          n126 = property on="Property Node" class="Ctl"(reference=w407, "Disabled"=u8 0) -> ()  [unwired: 1 in, 2 out]
                        }
                        frame "Left Wall Follow" {
                          # "All attributes are valid for this\noperation."
                          n127 = Index Array "Index Array"(array=w409, index=1) -> (element=w411:refnum<vi>)
                          n128 = property on="Property Node" class="Ctl"(reference=w411, "Disabled"=u8 0) -> ()  [unwired: 1 in, 2 out]
                        }
                        frame "Goto WayPoint" {
                          # "All attributes are valid for this\noperation."
                          n129 = Index Array "Index Array"(array=w413, index=1) -> (element=w415:refnum<vi>)
                          n130 = property on="Property Node" class="Ctl"(reference=w415, "Disabled"=u8 0) -> ()  [unwired: 1 in, 2 out]
                        }
                        frame "Circle" {
                          # "All attributes are valid for this\noperation."
                          n131 = Index Array "Index Array"(array=w417, index=1) -> (element=w419:refnum<vi>)
                          n132 = property on="Property Node" class="Ctl"(reference=w419, "Disabled"=u8 0) -> ()  [unwired: 1 in, 2 out]
                        }
                        frame "Right Wall Follow" {
                          # "All attributes are valid for this\noperation."
                          n133 = Index Array "Index Array"(array=w421, index=1) -> (element=w423:refnum<vi>)
                          n134 = property on="Property Node" class="Ctl"(reference=w423, "Disabled"=u8 0) -> ()  [unwired: 1 in, 2 out]
                        }
                        frame "Hunt" {
                          # "All attributes are valid for this\noperation."
                          n135 = Index Array "Index Array"(array=w425, index=1) -> (element=w427:refnum<vi>)
                          n136 = property on="Property Node" class="Ctl"(reference=w427, "Disabled"=u8 0) -> ()  [unwired: 1 in, 2 out]
                        }
                      }
                      n137 = local read "initialized MDF"() -> (w393:T4)
                    }
                    event "MissionDefFile": Mouse Up {
                      # "When the user is finished drawing, we complete the operation."
                      # "Finished Drawing"
                      n138 = event-data() -> ()  [unwired: 1 in, 3 out]
                      n139 = local write "Draw??"(FALSE ("Draw??")) -> ()
                      n140 = local read "initialized MDF"() -> (w430:T4)
                    }
                  }
                  "MissionDefFile" <- w303
                  "MDF_Original" <- w301
                  n141 = call "UpdateMDF.vi"("Index"=0, "MDF_In"=w301) -> ("MDF_Out"=→"MDF":T4)  [unwired: 9 in]
                }
                n142 = Wait (ms)(milliseconds to wait=u32 200) -> ()  [unwired: 1 out]
                "Way Point Index" <- 0 ("Boundary Point Index")
              }
              frame #1 {
                w434 = T8."AutoMode" ("Tab")
                # "Force \nnext \ncase\nto  be\nAutoMode"
                n143 = local write "Tab"(w434) -> ()
                n144 = local write "Exit Planning"(FALSE ("Exit Planning")) -> ()
              }
            }
          }
          frame "ManualMode" {
            # "Removing map shift register\nfixed memory leak?"
            # "Manual Steering by dashboard heading steering wheel\nand by speed slider"
            # "This mode lets \noperator directly\ndrive robot via\nthe ManualMode\ntabbed interface"
            n145 = while {
              shift-right: [w464] -> _
              shift-left: _ -> [w463]
              tunnel: w438 -> [w456]
              shift-right: [w453] -> _
              shift-left: _ -> [w452]
              tunnel: w436 -> [w450]
              stop <- w462 stop-if-true
              # "WhereAmI?"
              n146 = Get Date/Time In Seconds "GetMiissionCurrentTime"() -> (seconds since 1Jan1904=w457:timestamp)
              n147 = call "WhereForebrainPerception.vi"("Where? Midbrain"="WhereAmI?FromBase") -> ("Where? Forebrain"=→"Where? Manual":T6, "(xr,yr)"=w453:cluster{"X":dbl, "Y":dbl}, "Direction"=w442:dbl)  [unwired: 3 in, 1 out]
              "(xr,yr)" <- w453
              n148 = local read "ManualModeStop"() -> (w462:bool)
              n149 = To Double Precision Float(number=w457) -> (double precision float=w458:dbl)
              n150 = Greater Or Equal?(x=w442, y=181.0) -> (x >= y?=w447:bool)
              n151 = local read "Manual Heading"() -> (w454:i16)
              n152 = Subtract(x=w458, y=w456) -> (x-y=w459:dbl)
              n153 = Not(x=w463) -> (.not. x?=w464:bool)
              n154 = call "DrawRobot.vi"("(xr,yr) old"=w452, "(xr,yr) new"=w453, "2D Picture"=w450) -> ("new picture"=→"ManualMissionMap":picture)
              n155 = Divide(x=w459, y=60.0) -> (x/y=w461:dbl)
              "MissionTime" <- w461
              n156 = Subtract(x=w442, y=360.0) -> (x-y=w445:dbl)
              n157 = shared-variable "My Computer\\RobotBrainExLibrary.lvlib\\MissionTime"(w461) -> ()  [unwired: 1 in, 1 out]
              n158 = Select(t=w445, s=w447, f=w442) -> (s? t:f=w444:dbl)
              n159 = Bundle("Direction"=w444, "Manual Heading"=w454) -> (→"Heading":cluster{"Direction":dbl, "Manual Heading":i16})  [unwired: 1 in]
              n160 = Wait Until Next ms Multiple(millisecond multiple=u32 100 ("milliseconds to wait")) -> ()  [unwired: 1 out]
              "Where? 2" <- w463
            }
            n161 = while {
              shift-right: [w471] -> _
              shift-left: _ -> [w472]
              stop <- "ManualModeStop" stop-if-true
              # "WhatIsAroundMe?"
              n162 = local read "WhatAroundMeMap?"() -> (w466:cluster{"T":dbl, "Range":dbl, "Bearing":dbl}[])
              n163 = call "ProcessLidarData.vi"("WhatAroundMe?MM"=w466) -> ("Collision"=w467:bool, "data array [mag, phase (deg)]"=w468:cluster{"magnitude":dbl, "phase":dbl}[])
              "CollisionLight" <- w467
              n164 = Not(x=w472) -> (.not. x?=w471:bool)
              "MWhat?" <- w471
              n165 = call "SimLIDARPlot.vi"("data array [mag, phase (deg)]"=w468) -> ("SONAR"=→"ManualModeMapDAR":picture)  [unwired: 1 in]
              n166 = case shown="True" w467 {
                frame False {
                  # "No \nBeep"
                }
                frame True {
                  n167 = call <vilib>:"Beep.vi"("use system alert? (T)"=TRUE, "duration (msec)"=u32 1000, "frequency (Hz)"=u32 900) -> ()  [unwired: 9 in]
                }
              }
              n168 = Wait Until Next ms Multiple(millisecond multiple=u32 100 ("milliseconds to wait")) -> ()  [unwired: 1 out]
            }
            n169 = while {
              shift-right: [w496] -> _
              shift-left: _ -> [w495]
              stop <- w494 stop-if-true
              # "HowAmI?"
              n170 = local read "Battery\nVolts"() -> (w493:i16)
              n171 = local read "ManualModeStop"() -> (w494:bool)
              n172 = Not(x=w495) -> (.not. x?=w496:bool)
              n173 = Divide(x=w493, y=i16 1000) -> (x/y=→"Battery":dbl)
              n174 = Wait Until Next ms Multiple(millisecond multiple=u32 100 ("milliseconds to wait")) -> ()  [unwired: 1 out]
              "How? 2" <- w495
            }
            n175 = while {
              shift-right: [w490] -> _
              shift-left: _ -> [w489]
              stop <- w488 stop-if-true
              # "ForebrainAct"
              n176 = local read "E-Stop"() -> (w486:bool)
              n177 = local read "ManualModeStop"() -> (w488:bool)
              n178 = Select(t=0.0, s=w486, f="Manual Vel") -> (s? t:f=w483:dbl)
              n179 = To Word Integer(number=w483) -> (16bit integer=w481:i16)
              "Speed" <- w481
              n180 = local read "Send String"() -> (→"Send String to NXT":string)
              n181 = To Word Integer(number="Behavior Command") -> (16bit integer=w478:i16)
              n182 = local write "Upper Midbrain Active"("Upper Midbrain Active") -> ()
              n183 = local write "Mode"(w478) -> ()
              n184 = local write "Desired \nVelocity"(w481) -> ()
              n185 = local write "Local\nHeading"("Manual Heading") -> ()
              n186 = Not(x=w489) -> (.not. x?=w490:bool)
              n187 = Wait Until Next ms Multiple(millisecond multiple=u32 50 ("milliseconds to wait")) -> ()  [unwired: 1 out]
              "ActManual" <- w489
            }
            n188 = local read "ManualModeStop"() -> (w439:bool)
            n189 = case shown="True" w439 {
              tunnel: [TRUE ("s") w500] -> w441
              tunnel: [T8."ManualMode" ("Tab") w501] -> w440
              frame False {
              }
              frame True {
                # "Debounce tab for clean transition"
                n190 = flat-sequence {
                  tunnel: [w507] -> w501
                  tunnel: [TRUE ("s")] -> w500
                  frame #0 {
                    n191 = Wait (ms)(milliseconds to wait=u32 100) -> ()  [unwired: 1 out]
                  }
                  frame #1 {
                    w507 = T8."Startup&Shutdown" ("Tab")
                    # "Turn off\nVelocity\non \nExit"
                    n192 = local write "ManualModeStop"(FALSE ("ManualModeStop")) -> ()
                    n193 = local write "Desired \nVelocity"(i16 0 ("Desired \nVelocity")) -> ()
                    n194 = local write "Local\nHeading"(i16 0 ("Local\nHeading")) -> ()
                    n195 = local write "Mode"(i16 0 ("Mode")) -> ()
                    n196 = local write "Tab"(w507) -> ()
                  }
                }
              }
            }
          }
          frame "AutoMode" {
            n197 = flat-sequence {
              tunnel: w515 -> [_]
              tunnel: [w518] -> w513
              tunnel: w512 -> [w518]
              tunnel: w511 -> [w517]
              tunnel: [w517] -> w510
              tunnel: w509 -> [_]
              tunnel: w513 -> [w525]
              tunnel: w510 -> [w523]
              tunnel: [w602] -> w516
              tunnel: [FALSE ("s")] -> w514
              frame #0 {
                # "Run Robot\nbased on\nmission\ndefinition\nfile"
                n198 = local write "AutoMissionMap"(w517) -> ()
                n199 = while {
                  shift-right: [w521] -> _
                  shift-left: _ -> [w520]
                  stop <- "RunAutoMode" continue-if-true
                  # "Wait for Run\nbutton press\nbefore\nturning on\nAutoMode\nCode"
                  n200 = Not(x=w520) -> (.not. x?=w521:bool)
                  n201 = Wait Until Next ms Multiple(millisecond multiple=u32 100 ("milliseconds to wait")) -> ()  [unwired: 1 out]
                  "Ready" <- w520
                }
              }
              frame #1 {
                n202 = while {
                  shift-right: [w571] -> _
                  shift-left: _ -> [w562]
                  tunnel: w525 -> [w566]
                  shift-right: [w564] -> _
                  shift-left: _ -> [w565]
                  tunnel: w523 -> [w557]
                  stop <- w561 stop-if-true
                  # "WhereAmI?"
                  n203 = local read "WhereAmI?FromBase"() -> (w556:T6)
                  n204 = Get Date/Time In Seconds "GetMiissionCurrentTime"() -> (seconds since 1Jan1904=w567:timestamp)
                  n205 = call "WhereForebrainPerception.vi"("Where? Midbrain"=w556) -> ("(xr,yr)"=w564:cluster{"X":dbl, "Y":dbl}, "Direction"=w550:dbl)  [unwired: 3 in, 2 out]
                  "Robot Position" <- w564
                  n206 = local read "RunAutoMode"() -> (w561:bool)
                  n207 = Greater Or Equal?(x=w550, y=181.0) -> (x >= y?=w554:bool)
                  n208 = To Double Precision Float(number=w567) -> (double precision float=w568:dbl)
                  n209 = Subtract(x=w568, y=w566) -> (x-y=w569:dbl)
                  n210 = Not(x=w562) -> (.not. x?=w571:bool)
                  n211 = call "DrawRobot.vi"("(xr,yr) old"=w565, "(xr,yr) new"=w564, "2D Picture"=w557) -> ("new picture"=→"AutoMissionMap":picture)
                  n212 = local read "SteerAngle"() -> (w559:dbl)
                  n213 = Divide(x=w569, y=60.0) -> (x/y=w563:dbl)
                  "MissionTimeAuto" <- w563
                  n214 = Subtract(x=w550, y=360.0) -> (x-y=w552:dbl)
                  n215 = Select(t=w552, s=w554, f=w550) -> (s? t:f=w551:dbl)
                  n216 = shared-variable "My Computer\\RobotBrainExLibrary.lvlib\\MissionTime"(w563) -> ()  [unwired: 1 in, 1 out]
                  n217 = Bundle("Direction"=w551, "SteerAngle"=w559) -> (→"A Heading":cluster{"Direction":dbl, "SteerAngle":dbl})  [unwired: 1 in]
                  n218 = Wait Until Next ms Multiple(millisecond multiple=u32 50 ("milliseconds to wait")) -> ()  [unwired: 1 out]
                  "Where?" <- w562
                }
                n219 = while {
                  shift-right: [w592] -> _
                  shift-left: _ -> [w591]
                  shift-right: [w574] -> _
                  shift-left: 0.0 ("SteerAngle") -> [w587]
                  stop <- w594 stop-if-true
                  # "needs to put out heading in local coordinates"
                  # "Think"
                  n220 = Not(x=w591) -> (.not. x?=w592:bool)
                  n221 = Or(x="Pause", y="E-Stop") -> (x .or. y?=w578:bool)
                  n222 = local read "WhereAmI?FromBase"() -> (w590:T6)
                  n223 = local read "WhatAroundMeMap?"() -> (w589:cluster{"T":dbl, "Range":dbl, "Bearing":dbl}[])
                  n224 = local read "MDF"() -> (w580:T4)
                  n225 = call "GotoWaypoint.vi"("InhibitIn"=w578, "CurrentSteerAngle"=w587, "WhatAroundMe? Clean"=w589, "WhereAmI? Clean"=w590, "MDF In"=w580) -> ("BehCom"=→"Current Behavior":T7, "MDF Out"=w582:T4, "ActCommand"=→"WayPointAct":dbl[], "Vel"=w575:dbl, "SteerAngle"=w574:dbl)  [unwired: 1 in, 1 out]
                  "SteerAngle" <- w574
                  "A Speed" <- w575
                  n226 = To Long Integer(number=w575) -> (32bit integer=w576:i32)
                  n227 = To Long Integer(number=w574) -> (32bit integer=w573:i32)
                  n228 = local write "MDF"(w582) -> ()
                  n229 = local write "Desired \nVelocity"(w576) -> ()
                  n230 = local read "RunAutoMode"() -> (w594:bool)
                  n231 = local write "Local\nHeading"(w573) -> ()
                  n232 = local read "MDF_Original"() -> (w585:T4)
                  n233 = local read "MDF"() -> (w584:T4)
                  n234 = Select(t=w585, s="Rerun MDF", f=w584) -> (s? t:f=w581:T4)
                  n235 = local write "MDF"(w581) -> ()
                  n236 = Wait Until Next ms Multiple(millisecond multiple=u32 50 ("milliseconds to wait")) -> ()  [unwired: 1 out]
                  "Neo-C" <- w591
                }
                n237 = while {
                  shift-right: [w543] -> _
                  shift-left: _ -> [w545]
                  stop <- w542 stop-if-true
                  # "WhatIsAroundMe?"
                  n238 = local read "WhatAroundMeMap?"() -> (w539:cluster{"T":dbl, "Range":dbl, "Bearing":dbl}[])
                  n239 = call "ProcessLidarData.vi"("WhatAroundMe?MM"=w539) -> ("Collision"=w540:bool, "data array [mag, phase (deg)]"=w544:cluster{"magnitude":dbl, "phase":dbl}[])
                  "CollisionLight 2" <- w540
                  n240 = local read "RunAutoMode"() -> (w542:bool)
                  n241 = call "SimLIDARPlot.vi"("data array [mag, phase (deg)]"=w544) -> ("SONAR"=→"AutoModeLIDAR":picture)  [unwired: 1 in]
                  n242 = Not(x=w545) -> (.not. x?=w543:bool)
                  "What?" <- w543
                  n243 = case shown="True" w540 {
                    frame False {
                      # "No \nBeep"
                    }
                    frame True {
                      n244 = call <vilib>:"Beep.vi"("use system alert? (T)"=TRUE, "duration (msec)"=u32 1000, "frequency (Hz)"=u32 900) -> ()  [unwired: 9 in]
                    }
                  }
                  n245 = Wait Until Next ms Multiple(millisecond multiple=u32 50 ("milliseconds to wait")) -> ()  [unwired: 1 out]
                }
                n246 = while {
                  shift-right: [w537] -> _
                  shift-left: _ -> [w536]
                  stop <- w535 stop-if-true
                  # "HowAmI?"
                  n247 = local read "Battery\nVolts"() -> (w533:i16)
                  n248 = local read "RunAutoMode"() -> (w535:bool)
                  n249 = Not(x=w536) -> (.not. x?=w537:bool)
                  n250 = Divide(x=w533, y=i16 1000) -> (x/y=→"AutoBattery":dbl)
                  n251 = Wait Until Next ms Multiple(millisecond multiple=u32 80 ("milliseconds to wait")) -> ()  [unwired: 1 out]
                  "How?" <- w536
                }
                n252 = while {
                  shift-right: [w530] -> _
                  shift-left: _ -> [w529]
                  stop <- w528 stop-if-true
                  # "calculate desired heading.vi"
                  # "see calc desired\nheading"
                  # "convert to \noutputtin\nDesired v and\nlocal heading"
                  # "chnage arbiter to be -180 to 180"
                  # "Note:\nadd other beh to\narbiter"
                  # "ForebrainAct"
                  n253 = local read "WayPointAct"() -> (w527:dbl[])
                  n254 = local read "RunAutoMode"() -> (w528:bool)
                  n255 = Not(x=w529) -> (.not. x?=w530:bool)
                  n256 = call "ForebrainArbiter.vi"("WaypointInput"=w527) -> ("ForebrainActCom"=w526:dbl[])  [unwired: 14 in]
                  n257 = shared-variable "My Computer\\RobotBrainExLibrary.lvlib\\ActCommand"(w526) -> ()  [unwired: 1 in, 1 out]
                  n258 = Wait Until Next ms Multiple(millisecond multiple=u32 50 ("milliseconds to wait")) -> ()  [unwired: 1 out]
                  "Act" <- w529
                }
              }
              frame #2 {
                w602 = T8."Startup&Shutdown" ("Tab")
                # "Set robot Vel to 0"
                # "Reset latched run\nswitch"
                # "Force control to\nShutdown Case"
                n259 = shared-variable "My Computer\\RobotBrainExLibrary.lvlib\\ForebrainCom"(T9 {"VelCom"=0.0, "BehCom"=enum."OpenFieldTransit"} ("ForebrainCom")) -> ()  [unwired: 1 in, 1 out]
                n260 = local write "RunAutoMode"(TRUE ("RunAutoMode")) -> ()
                n261 = Initialize Array(0.0 ("element"), 90 ("dimension size")) -> (w598:dbl[])
                n262 = shared-variable "My Computer\\RobotBrainExLibrary.lvlib\\ActCommand"(w598) -> ()  [unwired: 1 in, 1 out]
                n263 = shared-variable "My Computer\\RobotBrainExLibrary.lvlib\\Xstart"(200.0 ("Xstart")) -> ()  [unwired: 1 in, 1 out]
                n264 = shared-variable "My Computer\\RobotBrainExLibrary.lvlib\\Ystart"(400.0 ("Ystart")) -> ()  [unwired: 1 in, 1 out]
                n265 = local write "Tab"(w602) -> ()
              }
            }
          }
          frame "Documentation" {
            # "Add:\n1) Blinking lights in each loop to show that they are running"
            # "This mode is just a static data flow picture of the ForeBrain"
            n266 = Wait (ms)(milliseconds to wait=u32 500) -> ()  [unwired: 1 out]
          }
          frame "DebugTHINK" {
            w612 = T8."Startup&Shutdown" ("Tab")
            # "Add:\n1) a button for each midbrain behavior to help in debugging\n2) graph of \"neural\" arbiter brain waves for each actuator\n3) a button for each forebrain behavior"
            # "Put code here in place of delay"
            # "Sends Tab Control\nback to Startup\ncase"
            n267 = Wait (ms)(milliseconds to wait=u32 5000) -> ()  [unwired: 1 out]
            n268 = local write "Tab"(w612) -> ()
          }
          frame "Basic AutoMode" {
            # "Index of Destination Point"
            # "Where am I?\nDraw robots current location on map"
            n269 = local read "Tug X"() -> (w652:i32)
            n270 = local read "Tug Y"() -> (w653:i32)
            n271 = Bundle("Tug X"=w652, "Tug Y"=w653) -> (w651:cluster{"Tug X":i32, "Tug Y":i32})  [unwired: 1 in]
            n272 = local read "Current Waypoint"() -> (w621:dbl)
            n273 = call "DrawRobot.vi"("(xr,yr) old"=w651, "(xr,yr) new"=w651, "2D Picture"=w650) -> ("new picture"=→"BAM Mission Map":picture)
            n274 = Array Size(array="Destinations Array") -> (size(s)=w618:i32[])
            n275 = Index Array(array="Destinations Array", index (row)=w621, index (col)=1 ("disabled index (col)")) -> (element=w627:i64)
            n276 = Index Array(array="Destinations Array", index (row)=w621, index (col)=0 ("index (row)")) -> (element=w629:i64)
            n277 = Index Array(array=w618, index=0) -> (element=→"Number Waypoints":i32)
            n278 = To Double Precision Float(number=w627) -> (double precision float=w628:dbl)
            n279 = To Double Precision Float(number=w629) -> (double precision float=w626:dbl)
            n280 = local read "WhereAmI?FromBase"() -> (w656:T6)
            n281 = Unbundle(w656) -> ("X"=w635:dbl, "Y"=w634:dbl, "Direction"=w655:dbl)  [unwired: 1 out]
            "Pixel X" <- w635
            "Pixel Y" <- w634
            "Direction" <- w655
            n282 = call "rudderAngle.vi"("BoatHeading"=w655, "YGoal"=w626, "XGoal"=w628, "Yboat"=w635, "Xboat"=w634) -> ("RudderAngle"=w641:dbl)  [unwired: 1 in, 2 out]
            n283 = call "NearWaypointTest.vi"("Yrobot"=w634, "Xrobot"=w635, "Ywaypoint"=w628, "Xwaypoiny"=w626) -> ("AtWaypoint"=w624:bool)  [unwired: 7 in]
            n284 = Select(t="Heading", s="Manual Override", f=w641) -> (s? t:f=w640:dbl)
            n285 = Select(t="Velocity", s="Manual Override", f=i16 8 ("t")) -> (s? t:f=w633:i16)
            n286 = local read "Number Waypoints"() -> (w615:i32)
            n287 = local read "Current Waypoint"() -> (w620:dbl)
            n288 = local read "Battery\nVolts"() -> (w648:i16)
            n289 = Increment(x=w620) -> (x+1=w623:dbl)
            n290 = Greater Or Equal?(x=w620, y=w615) -> (x >= y?=w614:bool)
            n291 = Divide(x=w648, y=1000) -> (x/y=→"Battery Level":dbl)
            n292 = Select(t=w623, s=w624, f=w620) -> (s? t:f=w625:dbl)
            n293 = local write "Current Waypoint"(w625) -> ()
            n294 = Select(t=i16 7, s=w614, f=w633) -> (s? t:f=w631:i16)
            n295 = local write "Local\nHeading"(w640) -> ()
            n296 = local write "Desired \nVelocity"(w631) -> ()
            n297 = local read "Tab"() -> (w644:T1)
          }
        }
        n298 = Not(x=w195) -> (.not. x?=w179:bool)
        "Robot Live" <- w179
      }
      n299 = while {
        tunnel: w58 -> [w161]
        tunnel: w57 -> [w160]
        tunnel: [w159] -> w55
        tunnel: [w158] -> w56
        shift-right: [w152] -> _
        shift-left: _ -> [w151]
        stop <- w162 continue-if-true
        w164 = 250  # timeout
        # "Finds and displays tugs position"
        # "runs continuously till program stops"
        # "Comminications with Base Station"
        # "receive string"
        # "If time out, post timeout and\nremove the timeout error"
        # "Read data from the port."
        n300 = Wait Until Next ms Multiple(millisecond multiple=u32 1) -> ()  [unwired: 1 out]
        n301 = UDP Read(connection ID=w161, timeout ms (25000)=w164, 8:w160) -> (data out=w153:string, error out=w165:errorcluster, 3:w158:refnum<k16>)  [unwired: 1 in, 2 out]
        "Base Station String" <- w153
        n302 = local write "Base Station data rec'd"(w153) -> ()
        n303 = Unbundle By Name(w165) -> ("code"=w168:i32)
        n304 = Equal?(x=w168, y=56) -> (x = y?=w166:bool)
        "BS Time Out?" <- w166
        n305 = case shown="True" w166 {
          tunnel: [w175 errorcluster {"status"=FALSE, "code"=0, "source"=""} ("error out")] -> w159
          tunnel: w165 -> [w175 _]
          frame False {
          }
          frame True {
          }
        }
        n306 = call "PC parse the data.vi"("Nav String"=w153, "Tug"="Tug letter") -> ("Buoy locations"=w157:cluster{"regular expression":string, i32, i32}[], "Tug Location"=w155:T14, "Valid?"=w156:bool)  [unwired: 1 out]
        "Valid ?" <- w156
        n307 = local write "Buoy locations"(w157) -> ()
        n308 = case shown="True" w156 {
          tunnel: w155 -> [_ w174]
          frame False {
            # "No \nchange"
          }
          frame True {
            # "New values from BaseStation"
            n309 = shared-variable "My Computer\\RobotBrainExLibrary.lvlib\\MissionTime"() -> (w173:dbl)  [unwired: 1 in, 1 out]
            n310 = Unbundle(w174) -> (w172:i32, w171:i32, w170:i32)  [unwired: 1 out]
            n311 = local write "Tug X"(w172) -> ()
            n312 = local write "Tug Y"(w171) -> ()
            n313 = local write "Tug H"(w170) -> ()
            n314 = Bundle(w173, w172, w171, w170) -> (w169:cluster{dbl, i32, i32, i32})  [unwired: 1 in]
            n315 = local write "WhereAmI?FromBase"(w169) -> ()
          }
        }
        n316 = local read "RunRobot"() -> (w162:bool)
        n317 = Not(x=w151) -> (.not. x?=w152:bool)
        "udp rate" <- w151
      }
      n318 = while {
        tunnel: w59 -> [_]
        stop <- w101 continue-if-true
        n319 = local read "Upper Midbrain Active"() -> (w100:bool)
        n320 = case shown="True" w100 {
          frame False {
            # "loop timimng \ncontrolled externally"
            # "Send commands to NXT"
            n321 = local read "Desired \nVelocity"() -> (w112:i16)
            n322 = local read "Local\nHeading"() -> (w111:i16)
            n323 = local read "Mode"() -> (w110:i16)
            n324 = case shown="2" w110 {
              tunnel: w112 -> [w115 w126 w133]
              tunnel: w111 -> [w114 w125 w134]
              tunnel: [w116 w121 w129] -> w104
              tunnel: i16 7 ("element") -> [w113 w122 w130]
              frame 0, Default {
                w117 = i16 0 ("element")
                n325 = Build Array(u8 91 ("element"), w113, w114, w115, i16 1 ("element"), w117, w117, w117, w117, w117, u8 93 ("element")) -> (w116:i16[])
              }
              frame 1 {
                w123 = i16 0 ("element")
                n326 = Build Array(u8 91 ("element"), w122, w125, w126, w123, i16 1 ("element"), w123, w123, w123, w123, u8 93 ("element")) -> (w121:i16[])
              }
              frame 2 {
                w131 = i16 0 ("element")
                n327 = Build Array(u8 91 ("element"), w130, w134, w133, w131, w131, i16 1 ("element"), w131, w131, w131, u8 93 ("element")) -> (w129:i16[])
              }
            }
            n328 = Select(t=u8[] [91, 7, 7, 7, 1, 0, 0, 0, 0, 0, 92], s="Soft E-Stop", f=w104) -> (s? t:f=w105:i16[])
            n329 = Add(x=w105, y=u8[] [0, 65, 65, 65, 65, 65, 65, 65, 65, 65, 0]) -> (x+y=w106:i16[])
            n330 = Byte Array To String(unsigned byte array=w106) -> (string=w103:string)
            n331 = local write "Send String"(w103) -> ()
          }
          frame True {
            n332 = local read "ManualModeStop"() -> (w138:bool)
            n333 = call "UpperMidbrain.vi"("SOFT E-STOP"=w138, "IR Servo"=u8 7) -> ("string"=w139:string)  [unwired: 9 in]
            n334 = local write "Send String"(w139) -> ()
          }
        }
        n335 = local read "RunRobot"() -> (w101:bool)
      }
      n336 = while {
        tunnel: w59 -> [_]
        stop <- w78 continue-if-true
        # "Receive information from NXT"
        n337 = local read "String Received"() -> (w83:string)
        n338 = Wait Until Next ms Multiple(millisecond multiple=u32 100) -> ()  [unwired: 1 out]
        n339 = String Subset(string=w83, offset (0)=1, length (rest)=1 ("length (rest)")) -> (substring=w82:string)
        n340 = case shown="\"N\"" w82 {
          tunnel: w83 -> [_ w85]
          frame Default {
          }
          frame "N" {
            # "0-15"
            # "Parse command \"N\""
            n341 = String Subset(string=w85, offset (0)=2, length (rest)=4 ("length (rest)")) -> (substring=w96:string)
            n342 = String Subset(string=w85, offset (0)=6, length (rest)=3 ("length (rest)")) -> (substring=w92:string)
            n343 = String Subset(string=w85, offset (0)=9, length (rest)=2 ("length (rest)")) -> (substring=w88:string)
            n344 = Decimal String To Number(string=w96) -> (number=w99:i32)  [unwired: 2 in, 1 out]
            n345 = Decimal String To Number(string=w92) -> (number=w91:i32)  [unwired: 2 in, 1 out]
            n346 = Decimal String To Number(string=w88) -> (number=w89:i32)  [unwired: 2 in, 1 out]
            n347 = To Word Integer(number=w99) -> (16bit integer=w95:i16)
            n348 = To Word Integer(number=w91) -> (16bit integer=w90:i16)
            n349 = To Long Integer(number=w89) -> (32bit integer=w84:i32)
            n350 = local write "LidarDist"(w90) -> ()
            n351 = local write "Battery\nVolts"(w95) -> ()
            n352 = local write "IR Index"(w84) -> ()
          }
        }
        n353 = local read "RunRobot"() -> (w78:bool)
      }
      n354 = while {
        stop <- w77 continue-if-true
        # "Run Simulated MapDAR"
        n355 = local read "Tug X"() -> (w75:i32)
        n356 = local read "Tug Y"() -> (w74:i32)
        n357 = local read "Tug H"() -> (w73:i32)
        n358 = Bundle "Bundle"("Tug X"=w75, "Tug Y"=w74, "Tug H"=w73) -> (w76:cluster{"Tug X":i32, "Tug Y":i32, "Tug H":i32})  [unwired: 1 in]
        n359 = call "HindbrainLIDAR_Sim.vi"("SubPosition"=w76) -> ("WhatAroundMe?"=→"WhatAroundMeMap?":cluster{"T":dbl, "Range":dbl, "Bearing":dbl}[])  [unwired: 10 in]
        n360 = local read "RunRobot"() -> (w77:bool)
      }
      "Current Waypoint" <- 0.0 ("Current Waypoint")
    }
    frame #2 {
      # "Close XBee Radio"
      # "Close UDP port"
      # "Realease LIDAR\nMemory"
      # "Reset Run \nSwitch"
      # "Shutdown Robot"
      n361 = call "Pixel_LIDAR_Close.vi"("error in (no error) 2"=w661, "Image"=w662) -> ()  [unwired: 1 in]
      n362 = local write "RunRobot"(TRUE ("RunRobot")) -> ()
      n363 = call "XB PC Close.vi"("error in (no error)"=w659, "VISA resource name"=w660) -> ()
      n364 = UDP Close(connection ID=w658, 8:w657) -> ()  [unwired: 2 out]
      "error out" <- w659
    }
  }
